vi "Rohde & Schwarz VNA Set Number of Points.vi"(6 "Channel":i8=1 min=1 max=99 step=1, 7 "Rohde & Schwarz VNA":T1, 8 "error in (no error)":errorcluster, 10 "Number Points":i32, 11 "VISA Resource Name":refnum<visa-resource-name>) -> (0 "error out":errorcluster, 3 "dup VISA Resource Name":refnum<visa-resource-name>)   [LabVIEW 2011]
doc: "This VI for the HP 8753B is used to read the number of stimulus points."
uses:
  TypeDefs/Rohde & Schwarz VNA Instrument Info.ctl
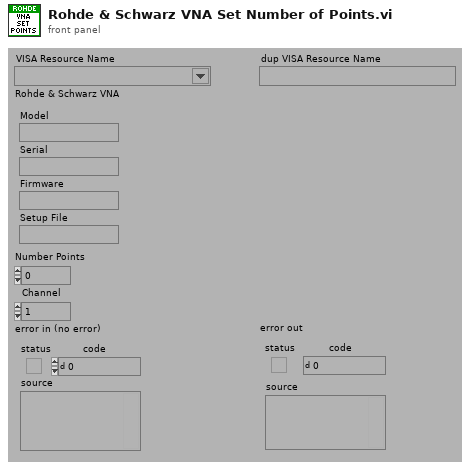
[diagram p1: front panel]
types:
  T1 = typedef "Rohde & Schwarz VNA Instrument Info.ctl" = cluster{"Model":string, "Serial":string, "Firmware":string, "Setup File":string}
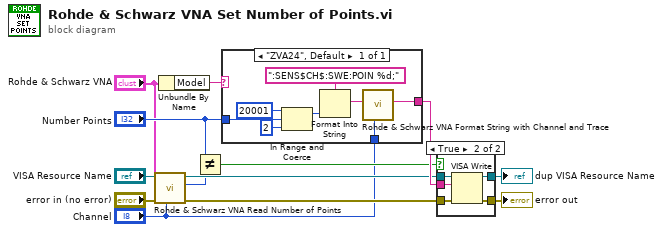
[diagram p0: block diagram]
diagram:
  n1 = call "Rohde & Schwarz VNA Read Number of Points.vi"("Channel"="Channel", "Rohde & Schwarz VNA"="Rohde & Schwarz VNA", "error in (no error)"="error in (no error)", "VISA Resource Name"="VISA Resource Name") -> ("error out"=w5:errorcluster, "Number Points"=w4:i32, "dup VISA Resource Name"=w6:refnum<visa-resource-name>)  [unwired: 5 out]
  n2 = Unbundle By Name("Rohde & Schwarz VNA") -> ("Model"=w1:string)
  n3 = Not Equal?(x="Number Points", y=w4) -> (x != y?=w9:bool)
  n4 = case shown="\"ZVA24\", Default" w1 {
    tunnel: [w15] -> w11
    tunnel: "Number Points" -> [w21]
    tunnel: "Channel" -> [w14]
    frame "ZVA24", Default {
      n5 = In Range and Coerce(upper limit=20001, x=w21, lower limit=2) -> (coerced(x)=w17:i32)  [unwired: 1 out]
      n6 = Format Into String(format string=":SENS$CH$:SWE:POIN %d;", w17) -> (resulting string=w16:string)  [unwired: 2 in, 1 out]
      n7 = call "Rohde & Schwarz VNA Format String with Channel and Trace.vi"("Channel"=w14, "String"=w16) -> ("String Out"=w15:string)  [unwired: 1 in, 6 out]
    }
  }
  n8 = case shown="True" w9 {
    tunnel: w6 -> [w23 w28]
    tunnel: w5 -> [w22 w27]
    tunnel: [w23 w26] -> w13
    tunnel: [w22 w25] -> w12
    tunnel: w11 -> [_ w24]
    frame False {
    }
    frame True {
      n9 = VISA Write(VISA resource name=w28, write buffer=w24, error in (no error)=w27) -> (VISA resource name out=w26:refnum<visa-resource-name>, error out=w25:errorcluster)  [unwired: 1 out]
    }
  }
  "dup VISA Resource Name" <- w13
  "error out" <- w12
